vi "RSZVB Set Number Of Readings.vi"(8 "error in (no error)":errorcluster {"code" format="%.0x"}, 9 "Number Of Readings (1)":i32=1, 10 "Channel (1)":i32=1, 11 "VISA session":refnum<visa-resource-name>) -> (0 "error out":errorcluster {"code" format="%.0x"}, 3 "dup VISA session":refnum<visa-resource-name>)   [LabVIEW 2011]
doc: "This VI sets a limit for the number of calibration sweeps in the source power calibration. The command is valid for all ports and external generators. Equivalent command: SOURce<Ch>:POWer<Pt>:CORRection:COLLect:AVERage[:COUNt]. \n\nRemote-control command(s):\nSOURce<Ch>:POWer<Pt>:CORRection:NREadings <readings>"
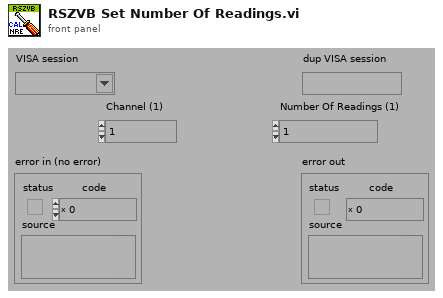
[diagram p1: front panel]
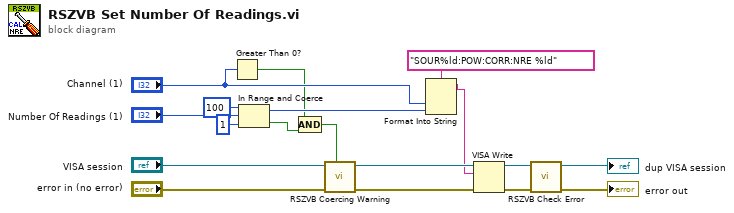
[diagram p0: block diagram]
diagram:
  n1 = Greater Than 0?(x="Channel (1)") -> (x > 0?=w3:bool)
  n2 = In Range and Coerce(upper limit=100, x="Number Of Readings (1)", lower limit=1) -> (coerced(x)=w4:i32, In Range?=w2:bool)
  n3 = Compound Arithmetic op=AND(w3, w2) -> (w1:bool)
  n4 = call "RSZVB Coercing Warning.vi"("In Range?"=w1, "error in (no error)"="error in (no error)", "VISA session"="VISA session") -> ("error out"=w17:errorcluster, "dup VISA session"=w18:refnum<visa-resource-name>)  [unwired: 7 in]
  n5 = Format Into String(format string="SOUR%ld:POW:CORR:NRE %ld", "Channel (1)", w4) -> (resulting string=w13:string)  [unwired: 2 in, 1 out]
  n6 = VISA Write(VISA resource name=w18, write buffer=w13, error in (no error)=w17) -> (VISA resource name out=w15:refnum<visa-resource-name>, error out=w16:errorcluster)  [unwired: 1 out]
  n7 = call "RSZVB Check Error.vi"("error in (no error)"=w16, "VISA session"=w15) -> ("error out"=→"error out":errorcluster, "dup VISA session"=→"dup VISA session":refnum<visa-resource-name>)  [unwired: 8 in]
